vi "Data Received.vi"(8 "error in (no error)":errorcluster, 10 "Updated Data":string, 11 "Send String in":refnum<class "Send String.lvclass">) -> (0 "error out":errorcluster, 3 "Send String out":refnum<class "Send String.lvclass">)   [LabVIEW 2020, in "Interface.lvlib" / "Send String.lvclass"]
uses:
  Send String.lvclass
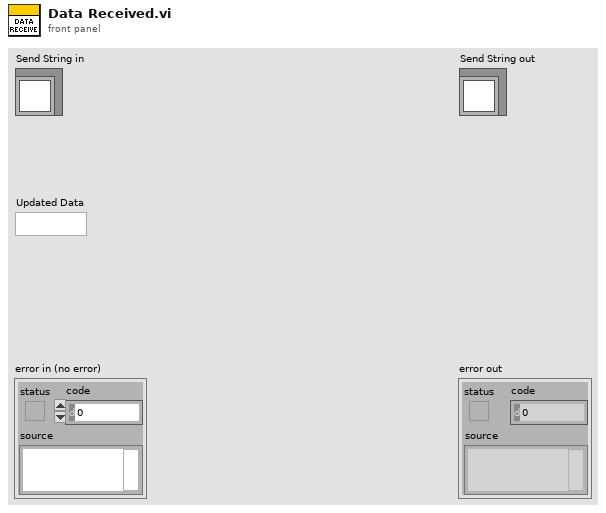
[diagram p1: front panel]
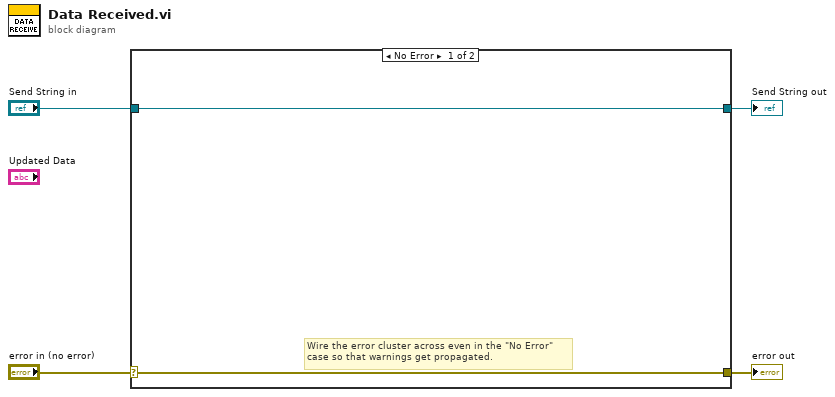
[diagram p0: block diagram]
diagram:
  n1 = case shown="No Error" "error in (no error)" {
    selector: "error in (no error)" -> [w5 w8]
    tunnel: [w5 w8] -> w3
    tunnel: [w6 w7] -> w1
    tunnel: "Send String in" -> [w6 w7]
    frame No Error {
      # "Wire the error cluster across even in the \"No Error\"\ncase so that warnings get propagated."
    }
    frame Error {
    }
  }
  "error out" <- w3
  "Send String out" <- w1
